vi "activity_info.vi"() -> ()   [LabVIEW 2009]
panel:
  in  "weight_2 sensor 3":dbl[][](array[numeric])
  in  "weight_2 sensor 2":dbl[][](array[numeric])
  in  "weight_2 sensor 1":dbl[][](array[numeric])
  in  "weight_1 sensor 3":dbl[][](array[numeric])
  in  "weight_1 sensor 2":dbl[][](array[numeric])
  in  "weight_1 sensor 1":dbl[][](array[numeric])
  out "Sensor 1":dbl[][](graph)
  in  "A":dbl[][](array[numeric])
  in  "D":dbl[][](array[numeric])
  in  "C":dbl[][](array[numeric])
  in  "B":dbl[][](array[numeric])
  in  "activity":dbl[][][](array[numeric])
  in  "weight_2":dbl[][](array[numeric])
  in  "weight_1":dbl[][](array[numeric])
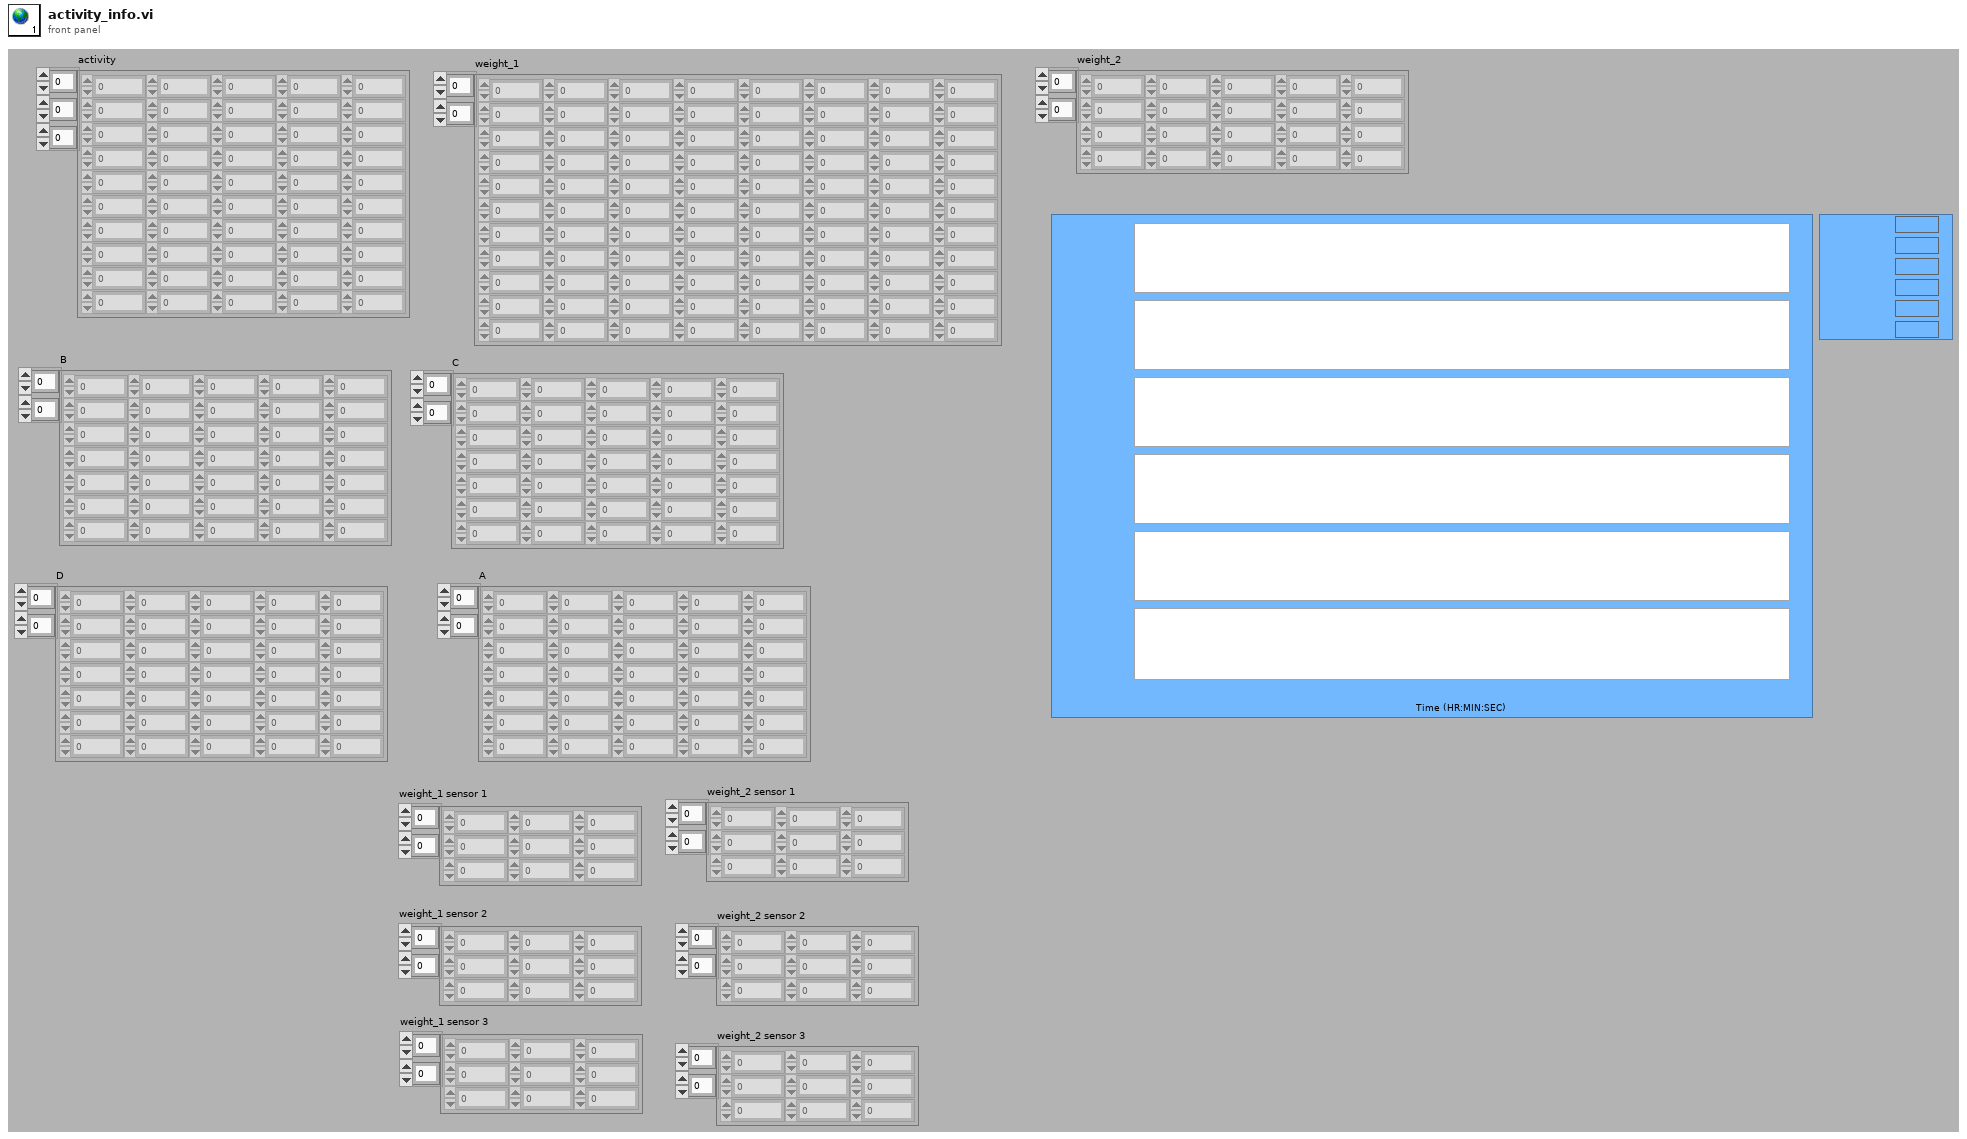
[diagram p1: front panel]
diagram:
